vi "jitterFunction.vi"(10 "jitterFraction":dbl, 11 "String in":string) -> (3 "String out":string, 4 "command":string)   [LabVIEW 2013]
doc: "This VI creates a string to define a jitter function, which can be used when plotting to separate values which otherwise would lie on top of each other."
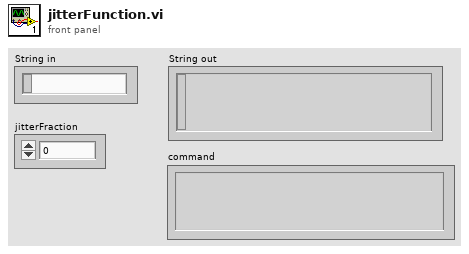
[diagram p1: front panel]
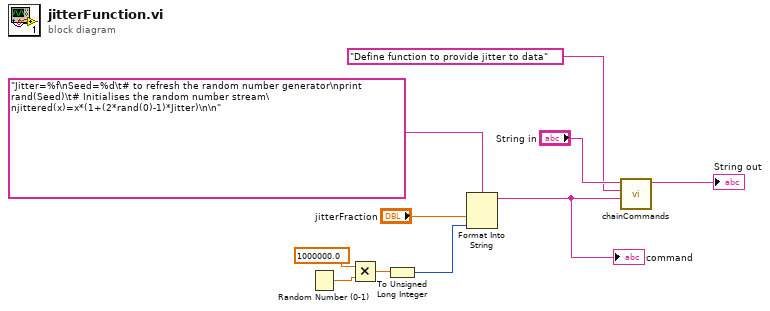
[diagram p0: block diagram]
diagram:
  n1 = Random Number (0-1)() -> (number: 0 to 1=w5:dbl)
  n2 = Multiply(x=1000000.0, y=w5) -> (x*y=w3:dbl)
  n3 = To Unsigned Long Integer(number=w3) -> (unsigned 32bit integer=w2:u32)
  n4 = Format Into String(format string="Jitter=%f\nSeed=%d\t# to refresh the random number generator\nprint rand(Seed)\t# Initialises the random number stream\njittered(x)=x*(1+(2*rand(0)-1)*Jitter)\n\n", "jitterFraction", w2) -> (resulting string=w6:string)  [unwired: 2 in, 1 out]
  "command" <- w6
  n5 = call "chainCommands.vi"("Command"=w6, "Comments"="Define function to provide jitter to data", "StringIn"="String in") -> ("StringOut"=→"String out":string)  [unwired: 8 in]
